vi "Number of Inf to NaN Conversions String.vi"(1 "# Inf >> NaN":i32) -> (0 "# inf >> NaN Conversion Sring":string)   [LabVIEW 2021, in "Arrays.lvlib"]
uses:
  Arrays.lvlib
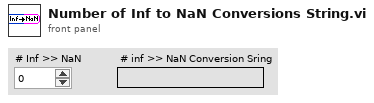
[diagram p1: front panel]
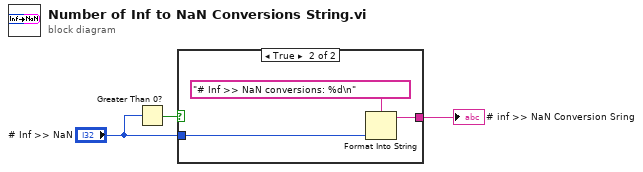
[diagram p0: block diagram]
diagram:
  n1 = Greater Than 0?(x="# Inf >> NaN") -> (x > 0?=w1:bool)
  n2 = case shown="True" w1 {
    tunnel: [_ w6] -> w3
    tunnel: "# Inf >> NaN" -> [_ w5]
    frame False {
    }
    frame True {
      n3 = Format Into String(format string="# Inf >> NaN conversions: %d\n", w5) -> (resulting string=w6:string)  [unwired: 2 in, 1 out]
    }
  }
  "# inf >> NaN Conversion Sring" <- w3
